vi "mono_gps_0.vi"(4 "error in":errorcluster, 5 "connection ID in":refnum<k5>) -> (0 "error out":errorcluster, 1 "gps_sample":T1, 3 "tcp_out":refnum<k5>)   [LabVIEW 2018]
uses:
  monoDrive.lvlib
panel:
  out "data out":string
  in  "vertical_acceleration":i32
  in  "horizontal_acceleration":u16
  in  "ego_speed":sgl
  in  "ego_yaw":sgl
  in  "forward_z":sgl
  in  "forward_y":sgl
  in  "forward_x":sgl
  in  "location_z":sgl
  in  "location_y":sgl
  in  "location_x":sgl
  in  "elevation":dbl format="%#_13g"
  in  "longitude":dbl format="%#_13g"
  in  "latitude":dbl format="%#_13g"
  in  "payload_length":u8
  in  "sensor_id":u16
  in  "MSG_POS_LLH":u16
  in  "preamble":u8
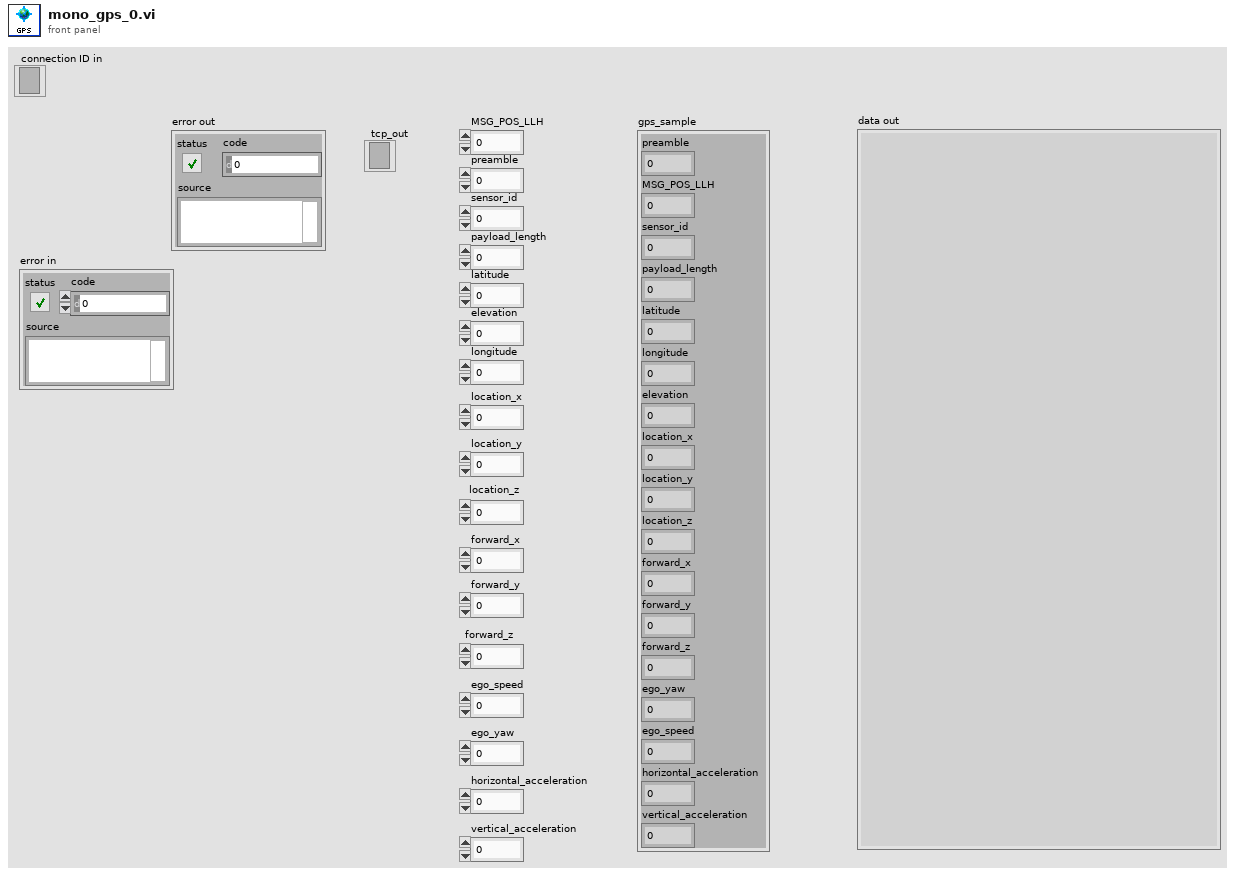
[diagram p1: front panel]
types:
  T1 = cluster{"preamble":u8, "MSG_POS_LLH":u16, "sensor_id":u16, "payload_length":u8, "latitude":dbl, "longitude":dbl, "elevation":dbl, "location_x":sgl, "location_y":sgl, "location_z":sgl, "forward_x":sgl, "forward_y":sgl, "forward_z":sgl, "ego_yaw":i32, "ego_speed":i32, "horizontal_acceleration":i32, "vertical_acceleration":i32}
  T2 = cluster{cluster{"length":u32, "time_stamp":u32, "game_time":sgl}, "data out":string}
  T3 = cluster{"preamble":u8, "MSG_POS_LLH":u16, "sensor_id":u16, "payload_length":u8, "latitude":dbl, "longitude":dbl, "elevation":dbl, "location_x":sgl, "location_y":sgl, "location_z":sgl, "forward_x":sgl, "forward_y":sgl, "forward_z":sgl, "ego_yaw":sgl, "ego_speed":sgl, "horizontal_acceleration":u16, "vertical_acceleration":i32}
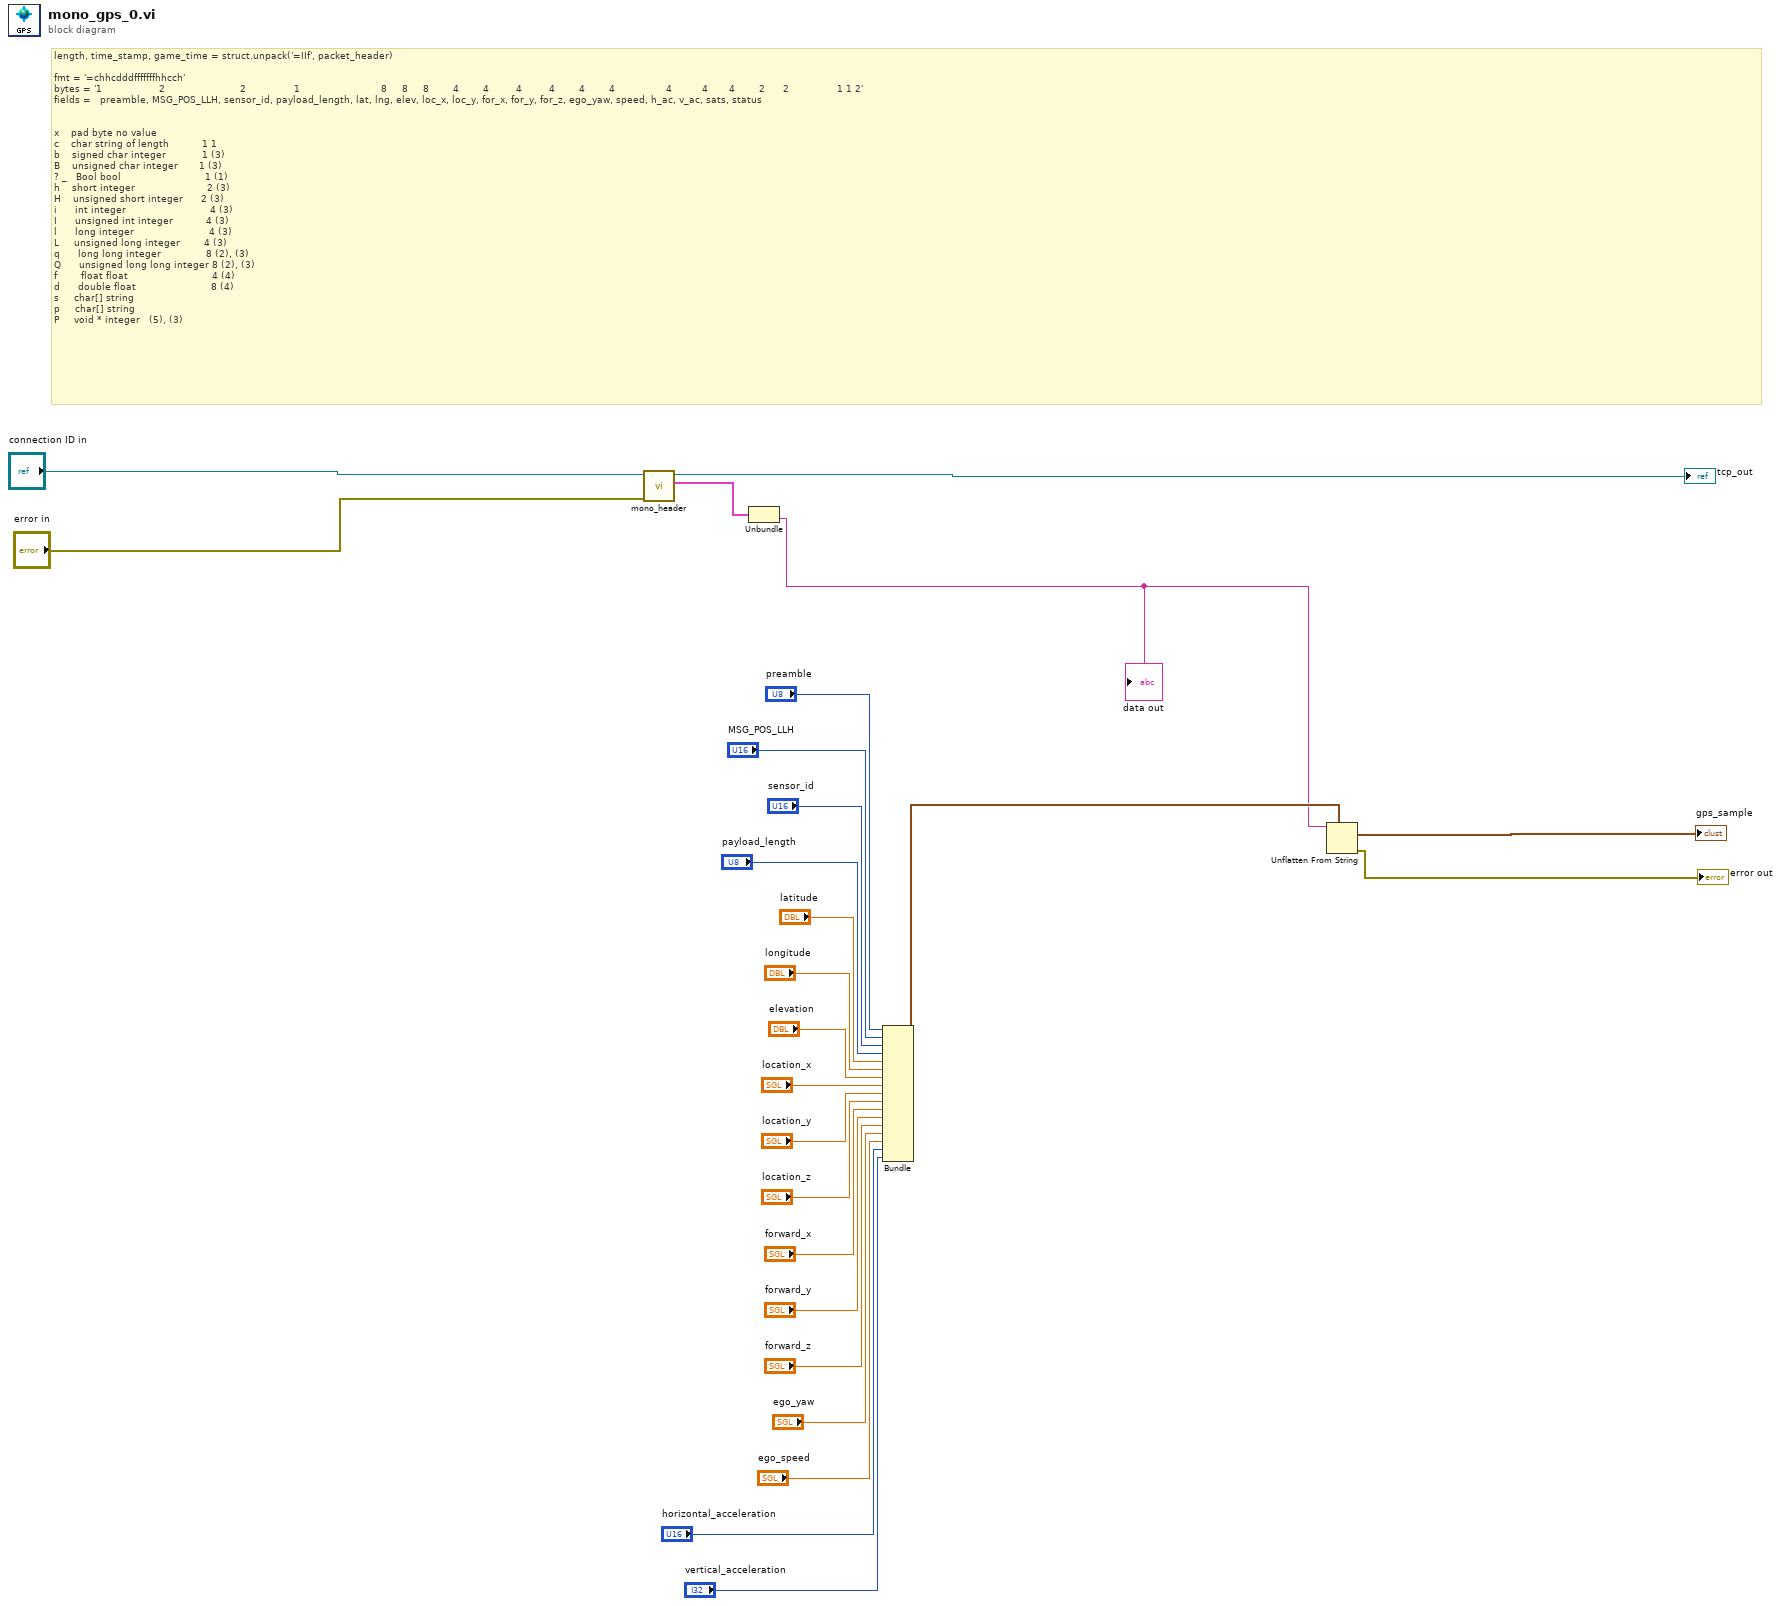
[diagram p0: block diagram]
diagram:
  # "length, time_stamp, game_time = struct.unpack('=IIf', packet_header)\n\nfmt = '=chhcdddfffffffhhcch'\nbytes = '1                   2                         2                1                           8     8     8        4        4         4         4        4        4                 4          4       4        2      2                1 1 2'\nfields =   preamble, MSG_POS_LLH, sensor_id, payload_length, lat, lng, elev, loc_x, loc_y, for_x, for_y, for_z, ego_yaw, speed, h_ac, v_ac, sats, status\n\n\nx\t   pad byte\tno value\t \t \nc\t   char\tstring of length           1\t1\t \nb\t   signed char\tinteger\t           1\t(3)\nB\t   unsigned char\tinteger\t      1\t(3)\n?\t_   Bool\tbool\t                           1\t(1)\nh\t   short\tinteger\t                       2\t(3)\nH\t   unsigned short\tinteger\t     2\t(3)\ni\t     int\tinteger\t                           4\t(3)\nI\t     unsigned int\tinteger\t          4\t(3)\nl     \tlong\tinteger\t                        4\t(3)\nL\t    unsigned long\tinteger\t       4\t(3)\nq     \tlong long\tinteger\t              8\t(2), (3)\nQ\t     unsigned long long\tinteger\t8\t(2), (3)\nf       \tfloat\tfloat\t                           4\t(4)\nd     \tdouble\tfloat\t                        8\t(4)\ns\t    char[]\tstring\t \t \np\t    char[]\tstring\t \t \nP\t    void *\tinteger\t \t(5), (3)"
  n1 = call "mono_header.vi"("error in"="error in", "connection ID"="connection ID in") -> ("sensor_sample"=w6:T2, "connection ID out"=→"tcp_out":refnum<k5>)  [unwired: 7 in, 1 out]
  n2 = Unbundle(w6) -> ("data out"=w3:string)  [unwired: 1 out]
  "data out" <- w3
  n3 = Bundle("preamble"="preamble", "MSG_POS_LLH"="MSG_POS_LLH", "sensor_id"="sensor_id", "payload_length"="payload_length", "latitude"="latitude", "longitude"="longitude", "elevation"="elevation", "location_x"="location_x", "location_y"="location_y", "location_z"="location_z", "forward_x"="forward_x", "forward_y"="forward_y", "forward_z"="forward_z", "ego_yaw"="ego_yaw", "ego_speed"="ego_speed", "horizontal_acceleration"="horizontal_acceleration", "vertical_acceleration"="vertical_acceleration") -> (w25:T3)  [unwired: 1 in]
  n4 = Unflatten From String(type=w25, binary string=w3) -> (value=→"gps_sample":T3, error out=→"error out":errorcluster)  [unwired: 3 in, 1 out]
